vi "RunTrajectoryCode.vi"(9 "HomeXY(pixels)":cluster{dbl, dbl}, 10 "TrajectoryImage":T1, 11 "Image":T1) -> (0 "error out":errorcluster, 2 "ImageOut":T1(plugin-control), 3 "TrajectoryImageOut":T1(plugin-control))   [LabVIEW 2017]
uses:
  <vilib>/vision/Image Controls.llb/IMAQ Image.ctl
panel:
  out "ChosenAngle":dbl
  out "Kicker XY":cluster{dbl, dbl}
  out "ChosenEnergy":dbl
  out "ChosenPathIdx":i32
  out "Puck":T2(array[cluster]) {"Position"."Y" format="%.2f"; "Position"."X" format="%.2f"}
  out "Players":T2(array[cluster]) {"Position"."Y" format="%.2f"; "Position"."X" format="%.2f"}
  out "Vertical Edges":T3(array[cluster]) {"Point2 (Real-World)"."Y" format="%.2f"; "Point2 (Real-World)"."X" format="%.2f"; "Point1 (Real-World)"."Y" format="%.2f"; "Point1 (Real-World)"."X" format="%.2f"; "Point2 (Pixels)"."Y" format="%.2f"; "Point2 (Pixels)"."X" format="%.2f"; "Point1 (Pixels)"."Y" format="%.2f"; "Point1 (Pixels)"."X" format="%.2f"}
  out "Horizontal Edges":T3(array[cluster]) {"Point2 (Real-World)"."Y" format="%.2f"; "Point2 (Real-World)"."X" format="%.2f"; "Point1 (Real-World)"."Y" format="%.2f"; "Point1 (Real-World)"."X" format="%.2f"; "Point2 (Pixels)"."Y" format="%.2f"; "Point2 (Pixels)"."X" format="%.2f"; "Point1 (Pixels)"."Y" format="%.2f"; "Point1 (Pixels)"."X" format="%.2f"}
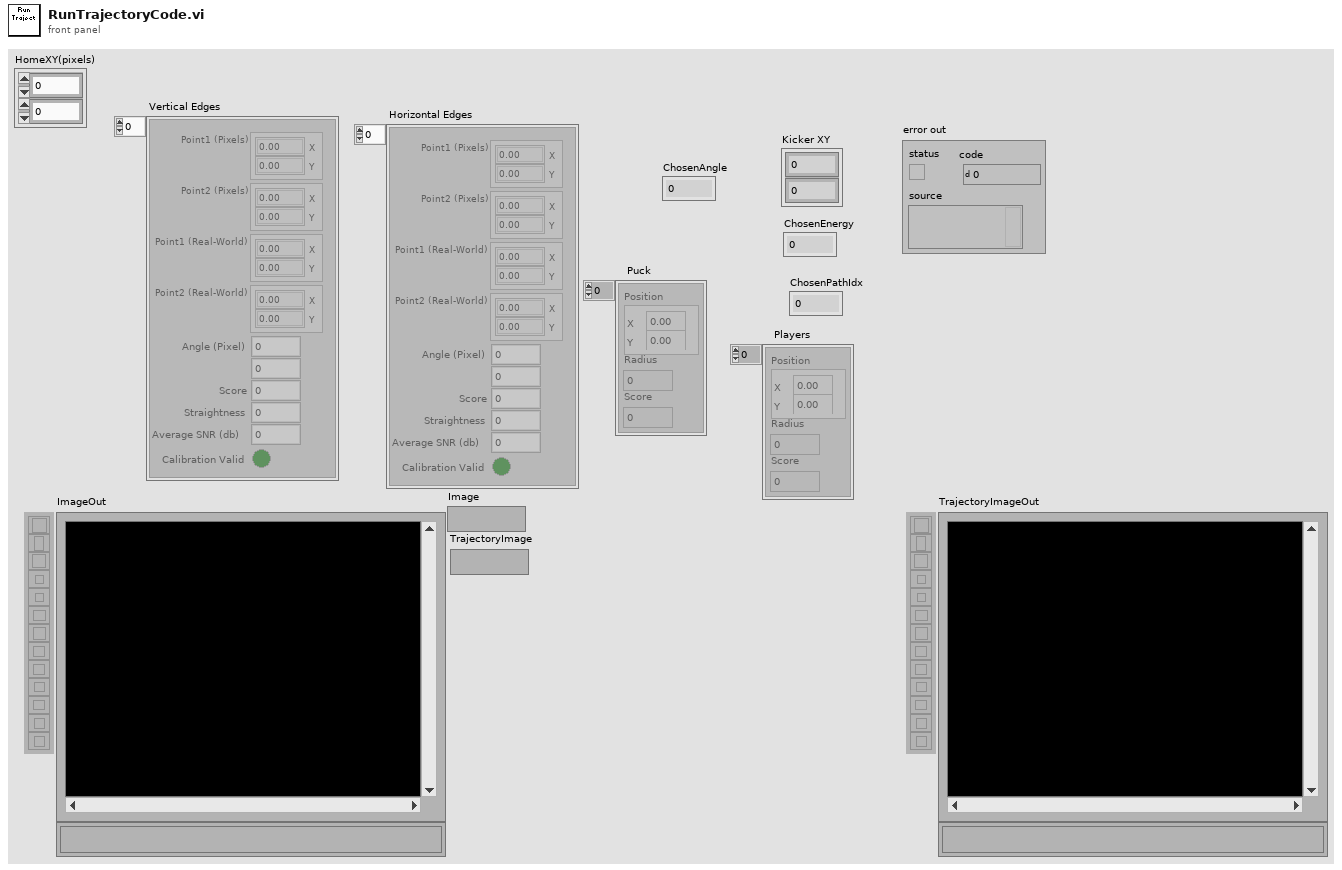
[diagram p1: front panel]
types:
  T1 = typedef "IMAQ Image.ctl" = refnum<image>
  T2 = cluster{"Position":cluster{"X":sgl, "Y":sgl}, "Radius":dbl, "Score":dbl}[]
  T3 = cluster{"Point1 (Pixels)":cluster{"X":sgl, "Y":sgl}, "Point2 (Pixels)":cluster{"X":sgl, "Y":sgl}, "Point1 (Real-World)":cluster{"X":sgl, "Y":sgl}, "Point2 (Real-World)":cluster{"X":sgl, "Y":sgl}, "Angle (Pixel)":dbl, "Angle (Real-World)":dbl, "Score":dbl, "Straightness":dbl, "Average SNR (db)":dbl, "Calibration Valid":bool}[]
  T4 = typedef "IMAQ Coordinate System" = cluster{"Reference System":cluster{"Origin":cluster{"X":sgl, "Y":sgl}, "Angle (deg)":sgl, "Axis Reference":u32}, "Measurement System":cluster{"Origin":cluster{"X":sgl, "Y":sgl}, "Angle (deg)":sgl, "Axis Reference":u32}}
  T5 = cluster{"Ptwx":dbl[], "Ptwy":dbl[], "Ptfx":dbl[], "Ptfy":dbl[], "DorR":i32[]}
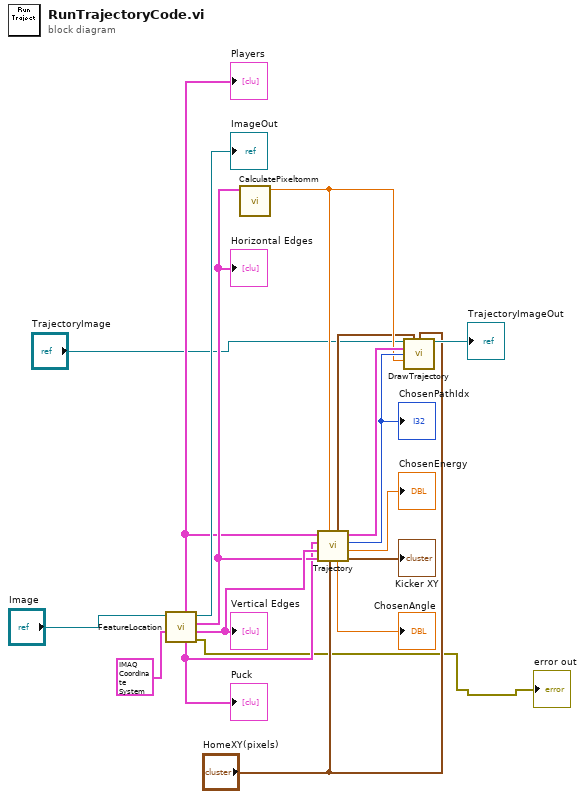
[diagram p0: block diagram]
diagram:
  n1 = call "FeatureLocation.vi"("Coordinate System"=T4 {"Reference System"={"Origin"={"X"=0.0, "Y"=0.0}, "Angle (deg)"=0.0, "Axis Reference"=0}, "Measurement System"={"Origin"={"X"=0.0, "Y"=0.0}, "Angle (deg)"=0.0, "Axis Reference"=0}}, "Image"="Image") -> ("error out"=→"error out":errorcluster, "Vertical Edges"=w18:T3, "Horizontal Edges"=w15:T3, "Image 2"=→"ImageOut":T1, "Puck"=w5:T2, "Players"=w6:T2)  [unwired: 4 in]
  "Horizontal Edges" <- w15
  "Vertical Edges" <- w18
  "Players" <- w6
  "Puck" <- w5
  n2 = call "CalculatePixeltomm.vi"("Horizontal Edges"=w15) -> ("Pixel/mm"=w9:dbl)  [unwired: 10 in]
  n3 = call "Trajectory.vi"("HomeXY(pixels)"="HomeXY(pixels)", "PixelmmRatio"=w9, "Horizontal Edges"=w15, "Vertical Edges"=w18, "Puck"=w5, "Players"=w6) -> ("Kicker XY"=→"Kicker XY":cluster{dbl, dbl}, "ChosenEnergy"=→"ChosenEnergy":dbl, "ChosenPathIdx"=w12:i32, "TrajectoryArray"=w14:T5, "Angle"=→"ChosenAngle":dbl, "PuckCentre"=w4:cluster{"PuckX":sgl, "PuckY":sgl})
  "ChosenPathIdx" <- w12
  n4 = call "DrawTrajectory.vi"("Image"="TrajectoryImage", "PuckCentre"=w4, "HomePoint(pixels)"="HomeXY(pixels)", "TrajectoryArray"=w14, "ChosenPath"=w12, "Pixel/mm"=w9) -> ("ImageOut"=→"TrajectoryImageOut":T1)  [unwired: 8 in, 1 out]
